vi "trial code new pid 02.vi"() -> ()   [LabVIEW 2025]
uses:
  <vilib>/Instr/_visa.llb/VISA Configure Serial Port (Instr).vi
  <vilib>/numeric/Random Number (Range) DBL.vi
panel:
  out "UNO":errorcluster
  in  "startup_cmd":dbl=400.0
  in  "min_amplitude":dbl
  in  "max_amplitude":dbl=1300.0
  in  "max_step_change":dbl=45.0
  in  "kd":dbl=40.0
  in  "ki":dbl=300.0
  in  "kp":dbl=1000.0
  out "prev_vc_cmd":dbl
  out "integral_accumulator_in":dbl
  out "prev_error":dbl
  in  "dt":dbl=0.05
  in  "STROKE":dbl[](array[numeric])=[0.1, 0.2, 0.3, 0.4, 0.5, 0.6, 0.7, 0.8, 0.9, 1.0, 1.1, 1.2]
  in  "1,2":dbl=1.1278
  in  "1.1":dbl=1.0761
  in  "1.0":dbl
  in  "0.9":dbl=0.9543
  in  "0.8":dbl
  in  "0.7":dbl=0.8122
  in  "0.6":dbl
  in  "0.5":dbl=0.639
  in  "0.4":dbl=0.5425
  in  "0.3":dbl=0.4226
  in  "0.2":dbl=0.2961
  in  "0.1":dbl=0.1677
  in  "calibration values":dbl[](array[numeric])=[0.1677, 0.2961, 0.4226, 0.5425, 0.639, 0.737, 0.8122, 0.864, 0.9543, 1.0177, 1.0761, 1.1278]
  in  "lower bound (0)":dbl
  in  "Stroke 2":dbl
  out "DUE":errorcluster
  out "Stroke RAW":dbl
  out "Stroke Tare":dbl
  in  "Boolean":bool
  in  "PID START COMMAND":bool
  in  "PID ACTUATE":bool
  in  "Stop 3":bool
  out "output Vpp":dbl
  in  "target_stroke":dbl=1.0
  in  "Stop 2":bool
  out "measured_stroke":dbl
  out "cof":dbl
  out "Friction":dbl
  out "pizo raw":dbl
  out "LVDT Peak":dbl
  out "LVDT MAX":dbl
  out "LVDT MIN":dbl
  in  "STROKE GAIN :":dbl=700.0 caption="Stroke Gain :"
  in  "Command":string
  in  "Stop":bool
  in  "Com Port 2":refnum<visa-resource-name>="COM9" caption="C2 :"
  out "Residual Uno 2":string
  out "Port 1 Error 2":errorcluster={"status"=TRUE, "code"=-1073807343, "source"="Property Node (arg 1) in VISA Configure Serial Port (Instr).vi->Winducom 2010--std ed hfrr-wo1768-V18.vi"}
  out "Uno":string
  out "Sps 4":dbl
  out "Port 1a 2":bool caption="Port 1 a"
  out "Error Uno 2":errorcluster={"status"=TRUE, "code"=-1073807343, "source"="Property Node (arg 1) in VISA Configure Serial Port (Instr).vi->Winducom 2010--std ed hfrr-wo1768-V18.vi"}
  out "Port 4":bool=TRUE caption="Port 1"
  in  "Re-initialize Port1 2":bool
  out "Residual Uno":string
  out "Port 1 Error":errorcluster={"status"=TRUE, "code"=-1073807343, "source"="Property Node (arg 1) in VISA Configure Serial Port (Instr).vi->Winducom 2010--std ed hfrr-wo1768-V18.vi"}
  out "due":string
  out "Sps 3":dbl
  out "Port 1a":bool caption="Port 1 a"
  out "Error Uno":errorcluster={"status"=TRUE, "code"=-1073807343, "source"="Property Node (arg 1) in VISA Configure Serial Port (Instr).vi->Winducom 2010--std ed hfrr-wo1768-V18.vi"}
  out "Port 3":bool=TRUE caption="Port 1"
  in  "Re-initialize Port1":bool
  out "FF buffer":dbl[](graph)
  in  "Com Port 1":refnum<visa-resource-name>="COM7" caption="C1 :"
  out "Test \nStatus":bool caption="Test Status"
types:
  T1 = cluster{"Read Heave and Surge":string, "Bytes at Heave Port":dbl, "Heave and Surge COM Port:":refnum<visa-resource-name>, "Com Port 2":refnum<visa-resource-name>, "Residual Due":string, "Heave COM Status 2":bool, "Heave COM Status":bool, "Port 2":bool, "Sway PPR":dbl, "Surge PPR":dbl, "Heave PPR":dbl, "Sway Pitch":dbl, "Surge Pitch":dbl, "Heave Pitch":dbl, "Sway Pulses/mm":dbl, "Surge Pulses/mm":dbl, "Heave Pulses/mm":dbl, "inner loop":dbl, "Read Heave and Surge 2":string, "String 36":string, "Write S":bool, "WriteCC1":string[], "Heave COM Loop":i32, "LastCom":string, "EXIT":bool, "Error Heave":errorcluster}
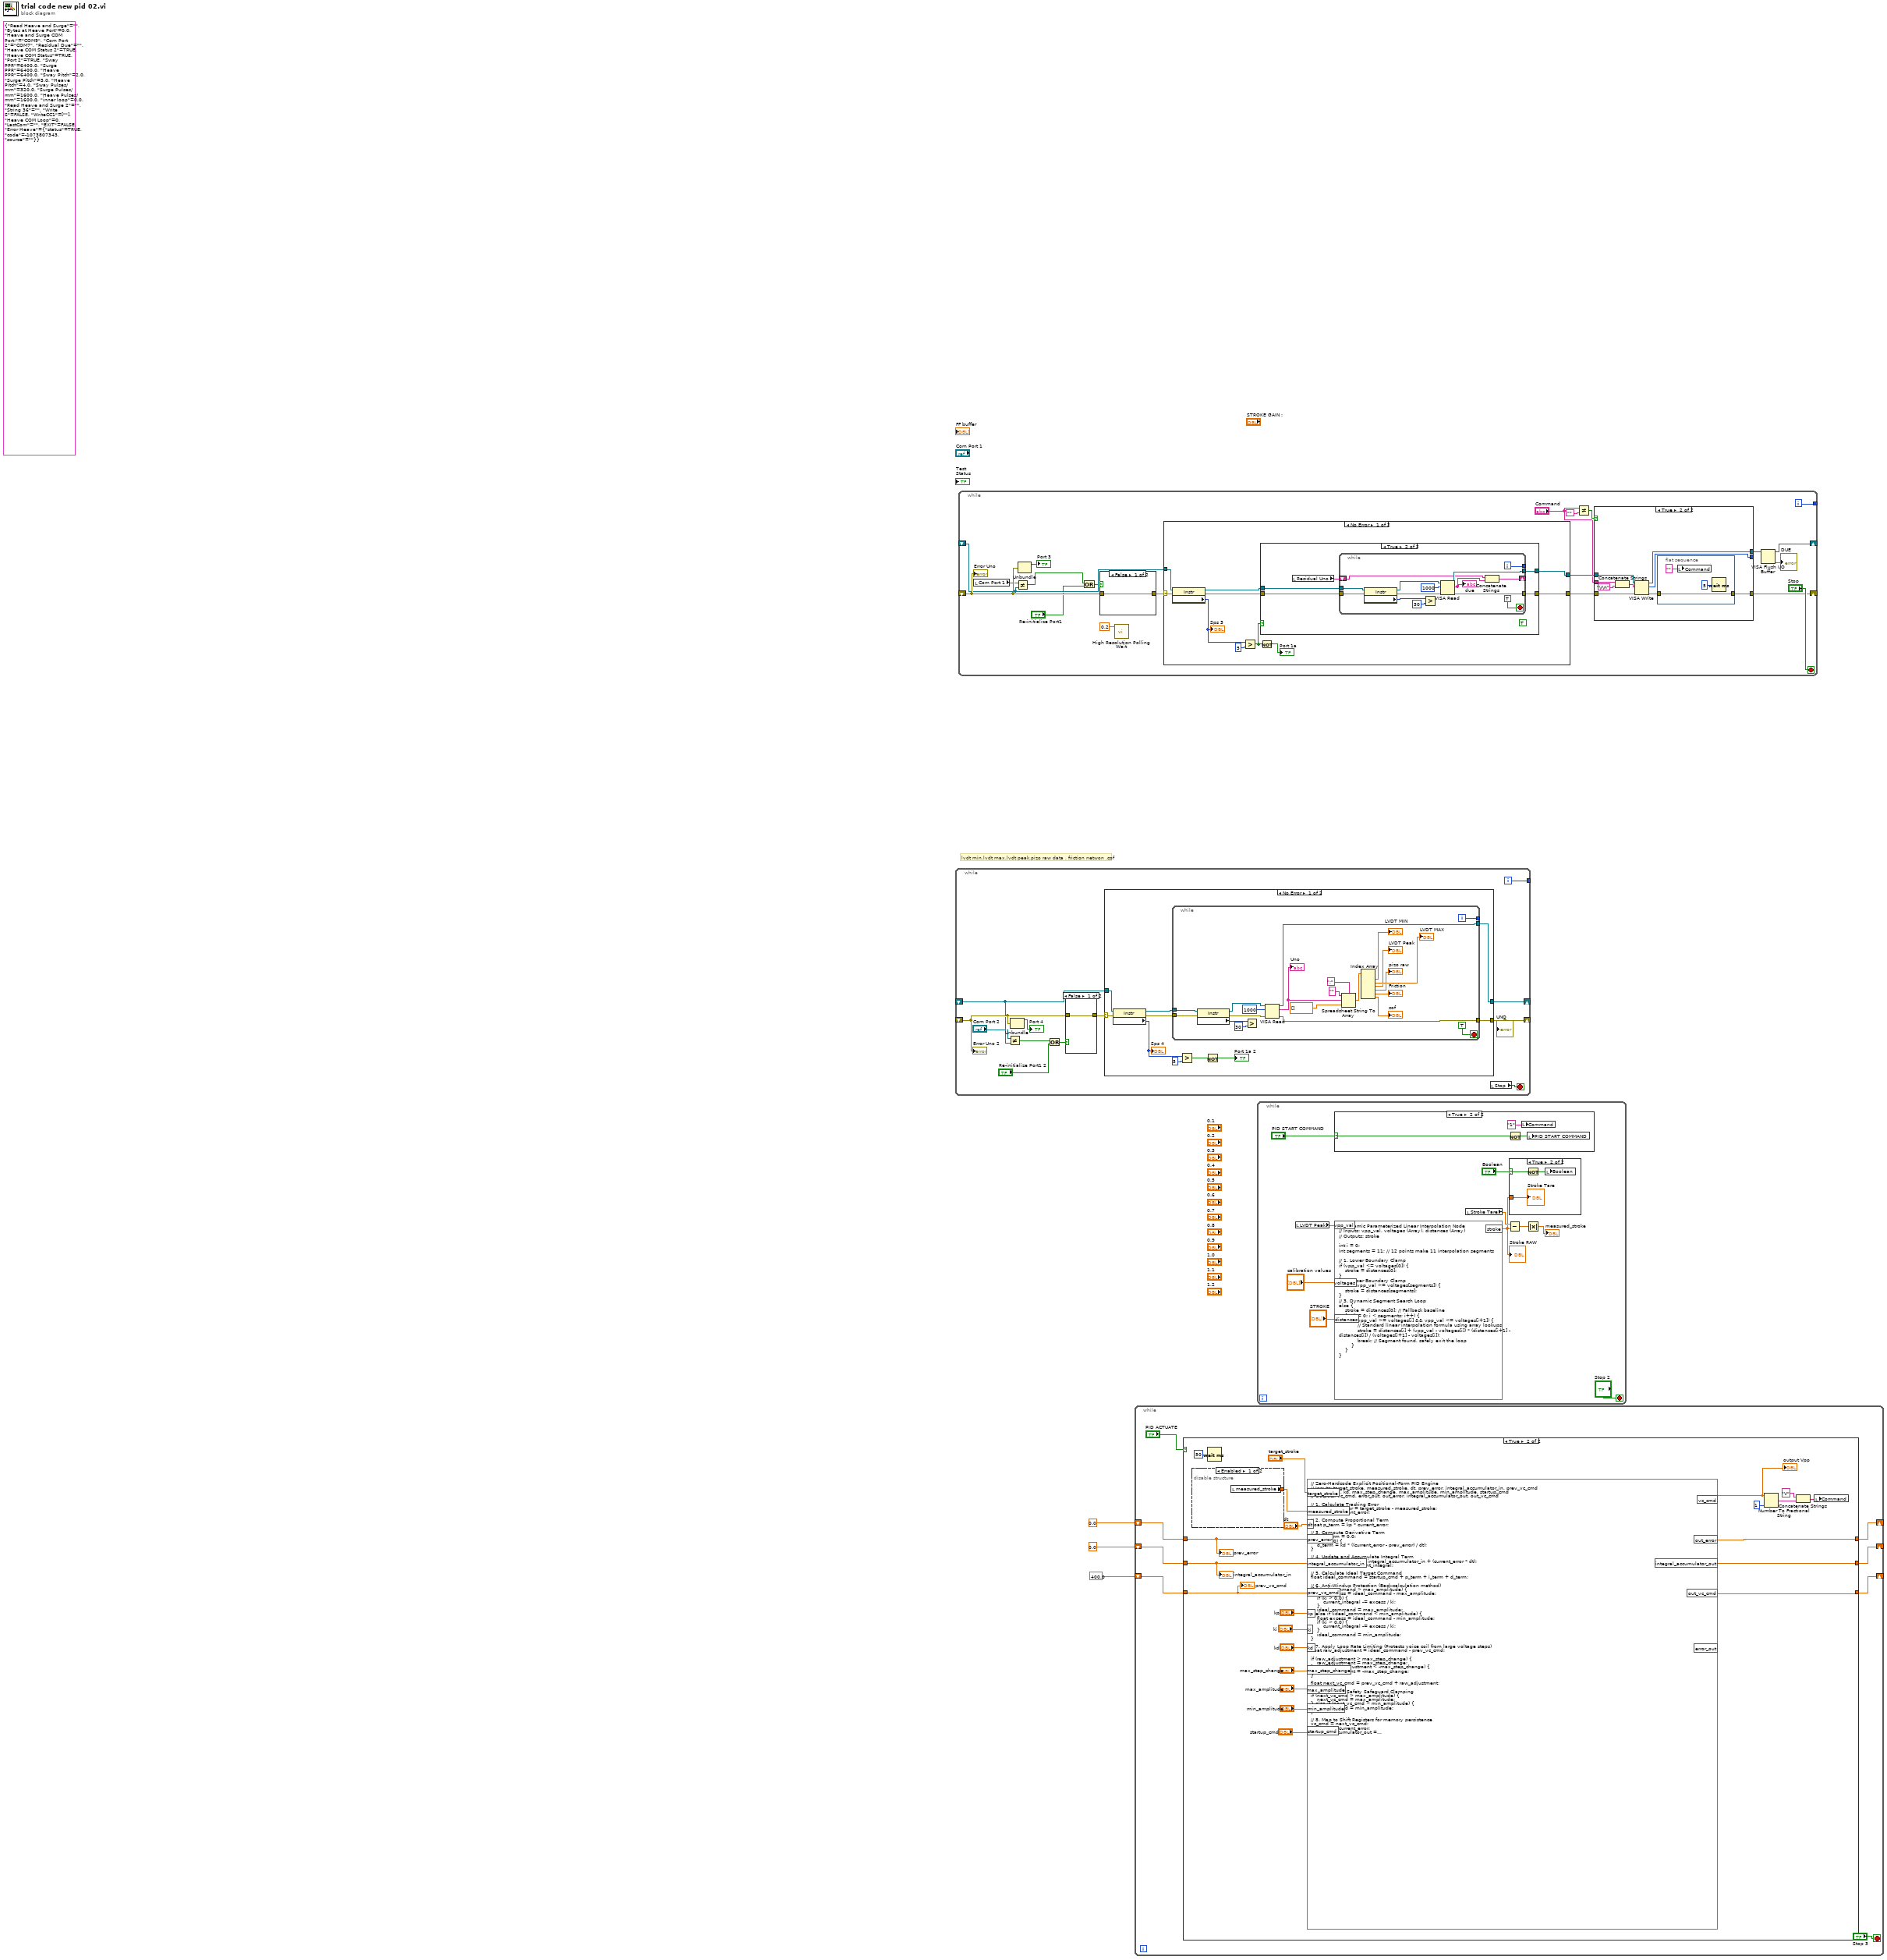
[diagram p0: block diagram]
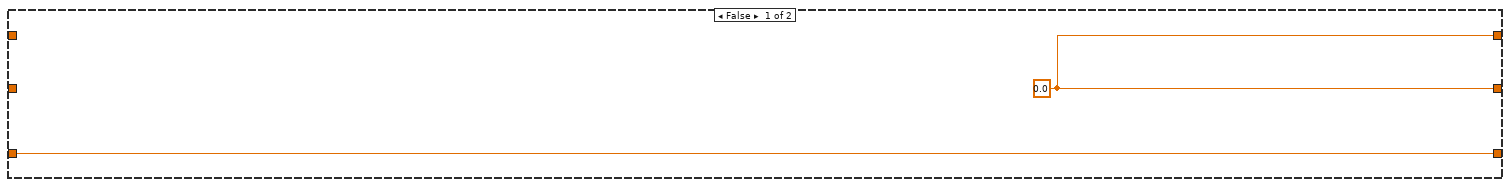
[diagram p2: hidden frame]
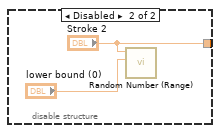
[diagram p3: hidden frame]
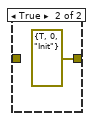
[diagram p6: hidden frame]
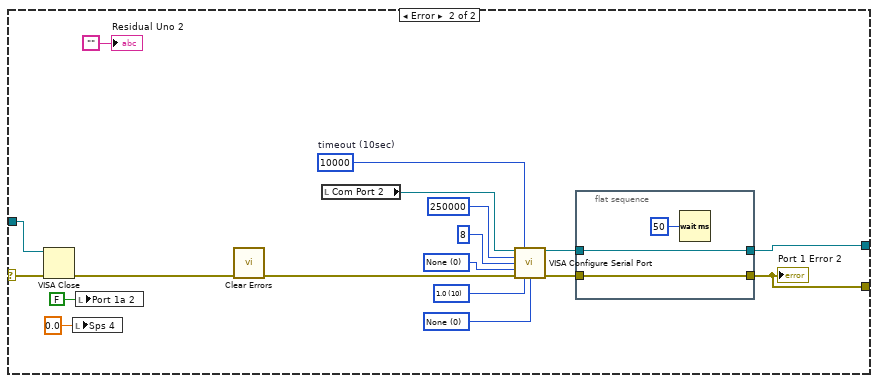
[diagram p7: hidden frame]
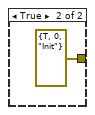
[diagram p9: hidden frame]
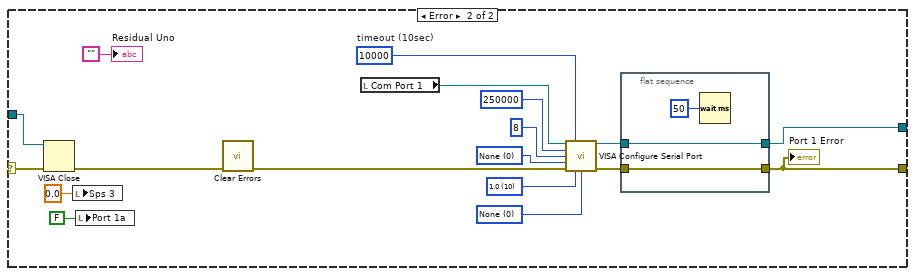
[diagram p11: hidden frame]
diagram:
  (unwired) T1 {"Read Heave and Surge"="", "Bytes at Heave Port"=0.0, "Heave and Surge COM Port:"="COM9", "Com Port 2"="COM7", "Residual Due"="", "Heave COM Status 2"=TRUE, "Heave COM Status"=TRUE, "Port 2"=TRUE, "Sway PPR"=6400.0, "Surge PPR"=6400.0, "Heave PPR"=6400.0, "Sway Pitch"=2.0, "Surge Pitch"=3.0, "Heave Pitch"=4.0, "Sway Pulses/mm"=320.0, "Surge Pulses/mm"=1600.0, "Heave Pulses/mm"=1600.0, "inner loop"=0.0, "Read Heave and Surge 2"="", "String 36"="", "Write S"=FALSE, "WriteCC1"=[""], "Heave COM Loop"=0, "LastCom"="", "EXIT"=FALSE, "Error Heave"={"status"=TRUE, "code"=-1073807343, "source"=""}}
  # "lvdt min,lvdt max,lvdt peak,pizo raw data , friction netwon ,cof"
  n1 = while {
    shift-right: [w15] -> _
    shift-left: _ -> [w10]
    shift-right: [w14] -> _
    shift-left: _ -> [w11]
    tunnel: [w13] -> _
    i -> [w13]
    stop <- w4 stop-if-true
    n2 = Not Equal?(x="Com Port 2", y=w10) -> (x != y?=w9:bool)
    n3 = Unbundle(w11) -> ("status"=→"Port 4":bool)  [unwired: 2 out]
    n4 = Or(x=w9, y="Re-initialize Port1 2") -> (x .or. y?=w7:bool)
    n5 = case shown="False" w7 {
      tunnel: [w16 errorcluster {"status"=TRUE, "code"=0, "source"="Init"} ("error out")] -> w8
      tunnel: w11 -> [w16 _]
      frame False {
      }
      frame True {
      }
    }
    n6 = case shown="No Error" w8 {
      selector: w8 -> [w24 w55]
      tunnel: [w27 w59] -> w15
      tunnel: [w26 w52] -> w14
      tunnel: w10 -> [w25 w57]
      frame No Error {
        n7 = property class="Instr"(reference=w25, error in=w24) -> (reference out=w22:refnum<visa-resource-name>, error out=w23:errorcluster, "Serial Settings:Number of Bytes at Serial Port"=w18:u32)
        "Sps 4" <- w18
        n8 = while {
          tunnel: [w47] -> w26
          tunnel: [w46] -> w27
          tunnel: w23 -> [w45]
          tunnel: w22 -> [w44]
          tunnel: [w42] -> _
          i -> [w42]
          stop <- TRUE stop-if-true
          n9 = property class="Instr"(reference=w44, error in=w45) -> (reference out=w49:refnum<visa-resource-name>, error out=w48:errorcluster, "Serial Settings:Number of Bytes at Serial Port"=w41:u32)
          n10 = Greater?(x=w41, y=u32 30) -> ()  [unwired: 1 out]
          n11 = VISA Read(VISA resource name=w49, byte count=u32 1000, error in (no error)=w48) -> (VISA resource name out=w46:refnum<visa-resource-name>, read buffer=w38:string, error out=w47:errorcluster)  [unwired: 1 out]
          "Uno" <- w38
          n12 = Spreadsheet String To Array(delimiter (Tab)=";", format string="", spreadsheet string=w38, array type (2D Dbl)=dbl[] []) -> (array=w35:dbl[])
          n13 = Index Array(array=w35) -> (element #1=→"LVDT MIN":dbl, element #2=→"LVDT MAX":dbl, element #3=→"LVDT Peak":dbl, element #4=→"pizo raw":dbl, element #5=→"Friction":dbl, element #6=→"cof":dbl)  [unwired: 6 in]
        }
        n14 = Greater?(x=w18, y=u32 5) -> (0:w20:bool)
        n15 = Not(x=w20) -> (.not. x?=→"Port 1a 2":bool)
      }
      frame Error {
        w65 = u16 0 items=["None", "XON/XOFF", "RTS/CTS", "XON/XOFF & RTS/CTS", "DTR/DSR", "XON/XOFF & DTR/DSR"] ("flow control (0:none)  2")
        w63 = u16 10 items=["1.0"=10, "1.5"=15, "2.0"=20] ("stop bits 2")
        w61 = u16 0 items=["None", "Odd", "Even", "Mark", "Space"] ("parity 2")
        w62 = u32 10000  # timeout (10sec)
        n16 = VISA Close(VISA resource name=w57, error in (no error)=w55) -> (error out=w58:errorcluster)
        n17 = local write "Sps 4"(0.0 ("Sps 4")) -> ()
        n18 = local write "Port 1a 2"(FALSE ("Port 1a")) -> ()
        n19 = call <vilib>:"Clear Errors.vi"("error in (no error)"=w58) -> ("error out"=w56:errorcluster)  [unwired: 5 in, 1 out]
        n20 = local read "Com Port 2"() -> (w50:refnum<visa-resource-name>)
        n21 = call-poly "VISA Configure Serial Port"("VISA resource name"=w50, "timeout (10sec)"=w62, "baud rate (9600)"=u32 250000 ("baud rate  2"), "data bits (8)"=u16 8 ("data bits  2"), "parity (0:none)"=w61, "error in (no error)"=w56, "stop bits (10: 1 bit)"=w63, "flow control (0:none)"=w65) -> ("VISA resource name out"=w66:refnum<visa-resource-name>, "error out"=w67:errorcluster)  [unwired: 6 in]
        n22 = flat-sequence {
          tunnel: w66 -> [w69]
          tunnel: w67 -> [w68]
          tunnel: [w69] -> w59
          tunnel: [w68] -> w52
          frame #0 {
            n23 = Wait (ms)(milliseconds to wait=u32 50) -> ()  [unwired: 1 out]
          }
        }
        "Residual Uno 2" <- ""
        "Port 1 Error 2" <- w52
      }
    }
    "UNO" <- w14
    n24 = local read "Stop"() -> (w4:bool)
    "Error Uno 2" <- w11
  }
  n25 = while {
    shift-right: [w72] -> _
    shift-left: _ -> [w86]
    shift-right: [w77] -> _
    shift-left: _ -> [w88]
    tunnel: [w90] -> _
    i -> [w90]
    stop <- "Stop" stop-if-true
    n26 = local read "Com Port 1"() -> (w87:refnum<visa-resource-name>)
    n27 = Not Equal?(x=w87, y=w86) -> (x != y?=w85:bool)
    n28 = Unbundle(w88) -> ("status"=→"Port 3":bool)  [unwired: 2 out]
    n29 = Or(x=w85, y="Re-initialize Port1") -> (x .or. y?=w83:bool)
    n30 = case shown="False" w83 {
      tunnel: [w105 errorcluster {"status"=TRUE, "code"=0, "source"="Init"} ("error out")] -> w84
      tunnel: w88 -> [w105 _]
      frame False {
      }
      frame True {
      }
    }
    n31 = call <vilib>:"High Resolution Polling Wait.vi"("seconds to wait"=0.2) -> ()  [unwired: 10 in, 1 out]
    n32 = case shown="No Error" w84 {
      selector: w84 -> [w113 w143]
      tunnel: [w116 w147] -> w78
      tunnel: [w115 w140] -> w79
      tunnel: w86 -> [w114 w145]
      frame No Error {
        n33 = property class="Instr"(reference=w114, error in=w113) -> (reference out=w111:refnum<visa-resource-name>, error out=w112:errorcluster, "Serial Settings:Number of Bytes at Serial Port"=w107:u32)
        "Sps 3" <- w107
        n34 = Greater?(x=w107, y=u32 5) -> (0:w109:bool)
        n35 = Not(x=w109) -> (.not. x?=→"Port 1a":bool)
        n36 = case shown="True" w109 {
          tunnel: w111 -> [w118 w122]
          tunnel: w112 -> [w117 w120]
          tunnel: [w117 w119] -> w115
          tunnel: [w118 w123] -> w116
          frame False {
          }
          frame True {
            (unwired) TRUE ("PAUSE")
            n37 = local read "Residual Uno"() -> (w121:string)
            n38 = while {
              tunnel: [w135] -> w119
              tunnel: [w134] -> w123
              tunnel: w120 -> [w133]
              tunnel: w122 -> [w132]
              tunnel: [w130] -> _
              shift-right: [w127] -> _
              shift-left: w121 -> [w128]
              i -> [w130]
              stop <- TRUE stop-if-true
              n39 = property class="Instr"(reference=w132, error in=w133) -> (reference out=w137:refnum<visa-resource-name>, error out=w136:errorcluster, "Serial Settings:Number of Bytes at Serial Port"=w129:u32)
              n40 = Greater?(x=w129, y=u32 30) -> ()  [unwired: 1 out]
              n41 = VISA Read(VISA resource name=w137, byte count=u32 1000, error in (no error)=w136) -> (VISA resource name out=w134:refnum<visa-resource-name>, read buffer=w124:string, error out=w135:errorcluster)  [unwired: 1 out]
              "due" <- w124
              n42 = Concatenate Strings(w128, w124) -> (w127:string)
            }
          }
        }
      }
      frame Error {
        w153 = u16 0 items=["None", "XON/XOFF", "RTS/CTS", "XON/XOFF & RTS/CTS", "DTR/DSR", "XON/XOFF & DTR/DSR"] ("flow control (0:none)  2")
        w151 = u16 10 items=["1.0"=10, "1.5"=15, "2.0"=20] ("stop bits 2")
        w149 = u16 0 items=["None", "Odd", "Even", "Mark", "Space"] ("parity 2")
        w150 = u32 10000  # timeout (10sec)
        n43 = VISA Close(VISA resource name=w145, error in (no error)=w143) -> (error out=w146:errorcluster)
        n44 = local write "Sps 3"(0.0 ("Sps 4")) -> ()
        n45 = local write "Port 1a"(FALSE ("Port 1a")) -> ()
        n46 = call <vilib>:"Clear Errors.vi"("error in (no error)"=w146) -> ("error out"=w144:errorcluster)  [unwired: 5 in, 1 out]
        n47 = local read "Com Port 1"() -> (w139:refnum<visa-resource-name>)
        n48 = call-poly "VISA Configure Serial Port"("VISA resource name"=w139, "timeout (10sec)"=w150, "baud rate (9600)"=u32 250000 ("baud rate  2"), "data bits (8)"=u16 8 ("data bits  2"), "parity (0:none)"=w149, "error in (no error)"=w144, "stop bits (10: 1 bit)"=w151, "flow control (0:none)"=w153) -> ("VISA resource name out"=w154:refnum<visa-resource-name>, "error out"=w155:errorcluster)  [unwired: 6 in]
        n49 = flat-sequence {
          tunnel: w154 -> [w157]
          tunnel: w155 -> [w156]
          tunnel: [w157] -> w147
          tunnel: [w156] -> w140
          frame #0 {
            n50 = Wait (ms)(milliseconds to wait=u32 50) -> ()  [unwired: 1 out]
          }
        }
        "Residual Uno" <- ""
        "Port 1 Error" <- w140
      }
    }
    n51 = Not Equal?(x="Command", y="") -> (x != y?=w74:bool)
    n52 = case shown="True" w74 {
      tunnel: w78 -> [w92 w97]
      tunnel: [w92 w101] -> w76
      tunnel: w79 -> [w91 w96]
      tunnel: [w91 w99] -> w77
      tunnel: "Command" -> [_ w95]
      tunnel: [_ w98] -> _
      frame False {
        # "DATA  WRITE LOOP"
      }
      frame True {
        n53 = Concatenate Strings(w95, "\r\n") -> (w94:string)
        n54 = VISA Write(VISA resource name=w97, write buffer=w94, error in (no error)=w96) -> (VISA resource name out=w101:refnum<visa-resource-name>, return count=w98:u32, error out=w100:errorcluster)
        n55 = flat-sequence {
          tunnel: w100 -> [w103]
          tunnel: [w103] -> w99
          frame #0 {
            n56 = local write "Command"("" ("command")) -> ()
            n57 = Wait (ms)(milliseconds to wait=u32 5) -> ()  [unwired: 1 out]
          }
        }
      }
    }
    n58 = VISA Flush I/O Buffer(VISA resource name=w76) -> (VISA resource name out=w72:refnum<visa-resource-name>, error out=→"DUE":errorcluster)  [unwired: 2 in]
    "Error Uno" <- w88
  }
  n59 = while {
    shift-right: [w160] -> _
    shift-left: 0.0 -> [w163]
    shift-right: [w159] -> _
    shift-left: 0.0 -> [w162]
    shift-right: [w161] -> _
    shift-left: 400.0 ("vc_cmd") -> [w166]
    stop <- "Stop 3" stop-if-true
    n60 = case shown="True" "PID ACTUATE" {
      tunnel: w166 -> [w168 w178]
      tunnel: w163 -> [_ w179]
      tunnel: w162 -> [_ w177]
      tunnel: [w168 w180] -> w161
      tunnel: [w167 w182] -> w160
      tunnel: [w167 w181] -> w159
      frame False {
        w167 = 0.0 ("error_out")
      }
      frame True {
        n61 = disable-structure shown="Enabled" {
          disable-tunnel: [w191 "Stroke 2"] -> w189
          frame Enabled {
            n62 = local read "measured_stroke"() -> (w191:dbl)
          }
          frame Disabled {
            n63 = call-poly <vilib>:"Random Number (Range).vi"("lower bound (0)"="lower bound (0)", "upper bound (100)"="Stroke 2") -> ()  [unwired: 9 in, 1 out]
          }
        }
        n64 = Wait (ms)(milliseconds to wait=u32 50) -> ()  [unwired: 1 out]
        n65 = formula code="// Zero-Hardcode Explicit Positional-Form PID Engine\n// Inputs: target_stroke, measured_stroke, dt, prev_error, integral_accumulator_in, prev_vc_cmd\n//         kp, ki, kd, max_step_change, max_amplitude, min_amplitude, startup_cmd\n// Outputs: vc_cmd, error_out, out_error, integral_accumulator_out, out_vc_cmd\n\n// 1. Calculate Tracking Error\nfloat current_error = target_stroke - measured_stroke;\nerror_out = current_error;\n\n// 2. Compute Proportional Term\nfloat p_term = kp * current_error;\n\n// 3. Compute Derivative Term\nfloat d_term = 0.0;\nif (dt > 0.0) {\n    d_term = kd * ((current_error - prev_error) / dt);\n}\n\n// 4. Update and Accumulate Integral Term\nfloat current_integral = integral_accumulator_in + (current_error * dt);\nfloat i_term = ki * current_integral;\n\n// 5. Calculate Ideal Target Command\nfloat ideal_command = startup_cmd + p_term + i_term + d_term;\n\n// 6. Anti-Windup Protection (Back-calculation method)\nif (ideal_command > max_amplitude) {\n    float excess = ideal_command - max_amplitude;\n    if (ki > 0.0) {\n        current_integral -= excess / ki;\n    }\n    ideal_command = max_amplitude;\n} else if (ideal_command < min_amplitude) {\n    float excess = ideal_command - min_amplitude;\n    if (ki > 0.0) {\n        current_integral -= excess / ki;\n    }\n    ideal_command = min_amplitude;\n}\n\n// 7. Apply Loop Rate Limiting (Protects voice coil from large voltage steps)\nfloat raw_adjustment = ideal_command - prev_vc_cmd;\n\nif (raw_adjustment > max_step_change) {\n    raw_adjustment = max_step_change;\n} else if (raw_adjustment < -max_step_change) {\n    raw_adjustment = -max_step_change;\n}\n\nfloat next_vc_cmd = prev_vc_cmd + raw_adjustment;\n\n// Final Output Safety Safeguard Clamping\nif (next_vc_cmd > max_amplitude) {\n    next_vc_cmd = max_amplitude;\n} else if (next_vc_cmd < min_amplitude) {\n    next_vc_cmd = min_amplitude;\n}\n\n// 8. Map to Shift Registers for memory persistence\nvc_cmd = next_vc_cmd;\nout_error = current_error;                     \nintegral_accumulator_out = current_integral;  \nout_vc_cmd = next_vc_cmd;"("target_stroke"="target_stroke", "measured_stroke"=w189, "dt"="dt", "integral_accumulator_in"=w179, "prev_error"=w177, "prev_vc_cmd"=w178, "kp"="kp", "ki"="ki", "kd"="kd", "max_step_change"="max_step_change", "max_amplitude"="max_amplitude", "min_amplitude"="min_amplitude", "startup_cmd"="startup_cmd") -> ("vc_cmd"=w187:dbl, "out_error"=w181:dbl, "integral_accumulator_out"=w182:dbl, "out_vc_cmd"=w180:dbl)  [unwired: 1 out]
        "output Vpp" <- w187
        n66 = Number To Fractional String(number=w187, precision (6)=i16 1) -> (F-format string=w185:string)  [unwired: 2 in]
        n67 = Concatenate Strings("V" ("string"), w185) -> (w183:string)
        n68 = local write "Command"(w183) -> ()
        "prev_error" <- w177
        "integral_accumulator_in" <- w179
        "prev_vc_cmd" <- w178
      }
    }
  }
  n69 = while {
    stop <- "Stop 2" stop-if-true
    n70 = local read "LVDT Peak"() -> (w203:dbl)
    n71 = case shown="True" "PID START COMMAND" {
      selector: "PID START COMMAND" -> [_ w209]
      frame False {
      }
      frame True {
        n72 = Not(x=w209) -> (.not. x?=w208:bool)
        n73 = local write "Command"("1" ("command")) -> ()
        n74 = local write "PID START COMMAND"(w208) -> ()
      }
    }
    n75 = formula code="// Dynamic Parameterized Linear Interpolation Node\n// Inputs: vpp_val, voltages (Array), distances (Array)\n// Outputs: stroke\n\nint i = 0;\nint segments = 11; // 12 points make 11 interpolation segments\n\n// 1. Lower Boundary Clamp\nif (vpp_val <= voltages[0]) {\n    stroke = distances[0];\n}\n// 2. Upper Boundary Clamp\nelse if (vpp_val >= voltages[segments]) {\n    stroke = distances[segments];\n}\n// 3. Dynamic Segment Search Loop\nelse {\n    stroke = distances[0]; // Fallback baseline\n    for (i = 0; i < segments; i++) {\n        if (vpp_val >= voltages[i] && vpp_val <= voltages[i+1]) {\n            // Standard linear interpolation formula using array lookups\n            stroke = distances[i] + (vpp_val - voltages[i]) * (distances[i+1] - distances[i]) / (voltages[i+1] - voltages[i]);\n            break; // Segment found, safely exit the loop\n        }\n    }\n}"("vpp_val"=w203, "voltages"="calibration values", "distances"="STROKE") -> ("stroke"=w198:dbl)
    "Stroke RAW" <- w198
    n76 = local read "Stroke Tare"() -> (w199:dbl)
    n77 = Subtract(x=w199, y=w198) -> (x-y=w197:dbl)
    n78 = case shown="True" "Boolean" {
      selector: "Boolean" -> [_ w206]
      tunnel: w198 -> [_ w204]
      frame False {
      }
      frame True {
        n79 = Not(x=w206) -> (.not. x?=w205:bool)
        n80 = local write "Boolean"(w205) -> ()
        "Stroke Tare" <- w204
      }
    }
    n81 = Absolute Value(x=w197) -> (abs(x)=→"measured_stroke":dbl)
  }
